vi "MagX Format Date.vi"(8 "error in":errorcluster, 11 "String":string) -> (0 "error out":errorcluster, 2 "Timestamp":timestamp, 3 "String out":string)   [LabVIEW 2025]
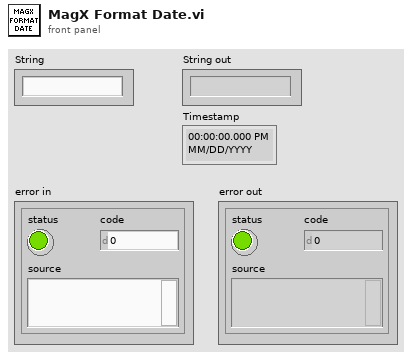
[diagram p1: front panel]
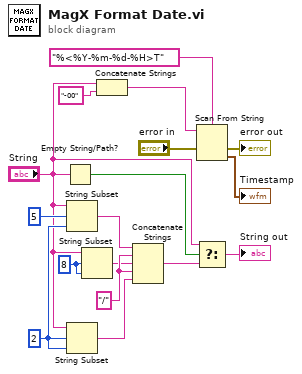
[diagram p0: block diagram]
diagram:
  w14 = "/" ("substring")
  w16 = 8 ("offset (0)")
  w15 = 2 ("offset (0)")
  n1 = Empty String/Path?(string/path="String") -> (empty?=w12:bool)
  n2 = String Subset(string="String", offset (0)=5, length (rest)=w15) -> (substring=w9:string)
  n3 = String Subset(string="String", offset (0)=w15, length (rest)=w15) -> (substring=w13:string)
  n4 = String Subset(string="String", offset (0)=w16, length (rest)=w16) -> (substring=w8:string)
  n5 = Concatenate Strings("String", "-00" ("string")) -> (w2:string)
  n6 = Concatenate Strings(w9, w14, w8, w14, w13) -> (w11:string)
  n7 = Scan From String(format string="%<%Y-%m-%d-%H>T", input string=w2, error in="error in") -> (error out=→"error out":errorcluster, output 1=→"Timestamp":timestamp)  [unwired: 2 in, 2 out]
  n8 = Select(t="String", s=w12, f=w11) -> (s? t:f=→"String out":string)
